vi "CommunicationTool - 副本.vi"(0 "VISA资源名称":refnum<visa-resource-name>="COM1", 1 "SN":string, 5 "通信协议名称":string, 7 "Slot":T1, 9 "DelayTime":u32=1000, 11 "error in":errorcluster, 12 "Debug":bool) -> (3 "字符串数值":bool=TRUE, 4 "响应":string="ÿÿÿÿÿÿÿÿÿÿÿÿÿÿÿÿÿÿÿÿÿÿÿÿÿÿÿ", 6 "反馈结果":bool, 10 "CMD":string, 14 "data":string, 15 "error out":errorcluster)   [LabVIEW 2013]
doc: "本范例根据用户指示，对串口执行读写操作。范例运行时可按下“写入”或“读取”按钮，以及修改“读数”。\n\n设置的串口参数必须匹配连接仪器或设备的参数。本范例中，“读数”参数可指定串口读取的字节数。如端口字节超过指定的字节数，超出部分将不会被读取。如端口字节数少于指定的字节数，将返回超时错误。\n\n本范例可扩展流控制选项以包括XON和XOFF，从而允许用户选择控制字符。同时，用户可启用或禁用中止符。部分设备需要通过终止符确定命令字符串的结束位置。部分设备将发送终止符以说明待读取数据的末端。本范例演示了缓冲区中检测到终止符时，结束“读取”操作或添加终止符至“写入”数据末端的方法。"
uses:
  SystemCode/SysControl/Slot.ctl
  <vilib>/Utility/NIReport.llb/NI_report.lvclass
  C:/Program Files/National Instruments/LabVIEW 2013/examples/Instrument IO/Serial/support/Serial - Settings.ctl
  SourceCode/GlobalValue.vi
  <vilib>/Utility/error.llb/Error Cluster From Error Code.vi
  <vilib>/addons/_office/excel.llb/Excel Get Data ([str]).vi
  <vilib>/Instr/_visa.llb/VISA Configure Serial Port (Instr).vi
  <vilib>/ErrorRing/Error Ring.xnode
  <vilib>/addons/_office/NI_ReportGenerationToolkit.lvlib
  <vilib>/Utility/NIReport.llb/Excel/NI_Excel.lvclass
panel:
  out "SerNO":string
  out "硬件版本":string
  out "终端ID":string
  out "CCID":string="PASS"
  out "生产日期":string
  out "字符串":string
  out "x-y":u32
  out "已删除的部分":u8[](array[numeric]) format="%x"
  out "读取缓冲区":string
  out "数据Hex":string[](array[string])
  out "数据ASCII":string[](array[string])
  out "数据类型":string[](array[string])
  in  "命令列表":u16(ring)=17 items=["启动自动化测试", "查询版本", "退出自动化测试", "进入待机模式", "进入工作模式", "查询ACC状态", "GPS定位查询", "GPS定位时间", "GPS可见星数", "3G通信自检", "3G信号强度", "查询网络状态", "拨号", "查询通话状态", "挂断", "外部Flash测试", "查询BAT7.2V_DET电压", "查询BAT_DET状态", "查询ANT1_0状态", "BATVCC_CTL输出低电平", "BATVCC_CTL输出高电平", "CHARGE_CTL输出低电平", "CHARGE_CTL输出高电平", "查询CHARGE_WAKE状态", "3G_PWR_CTL输出低电平", "3G_PWR_CTL输出高电平", "3G_RST输出低电平", "3G_RST输出高电平", "查询ANT1_S状态", "GPS_PWREN输出低电平", "GPS_PWREN输出高电平", "CAN通信接收", "CAN通信发送", "重启", "U_CTL输出低电平", "U_CTL输出高电平", "OBD_CTL输出低电平", "OBD_CTL输出高电平", "OBD_STB输出低电平", "OBD_STB输出高电平", "3G_EN输出低电平", "3G_EN输出高电平", "写入五菱主机条码", "写入主机条码", "读出五菱主机条码", "读出主机条码", "写入生产日期", "读出生产日期", "读出CCID", "写入终端ID", "读出终端ID", "写入硬件版本", "读出硬件版本", "查看TBC文件"]
  out "Write":bool
  out "Read":bool
  out "ConfigPath":string="C:\\Users\\dell\\Desktop\\ExcelReport.vi"
  out "Data":string
  out "DataType":string
  out "命令":string
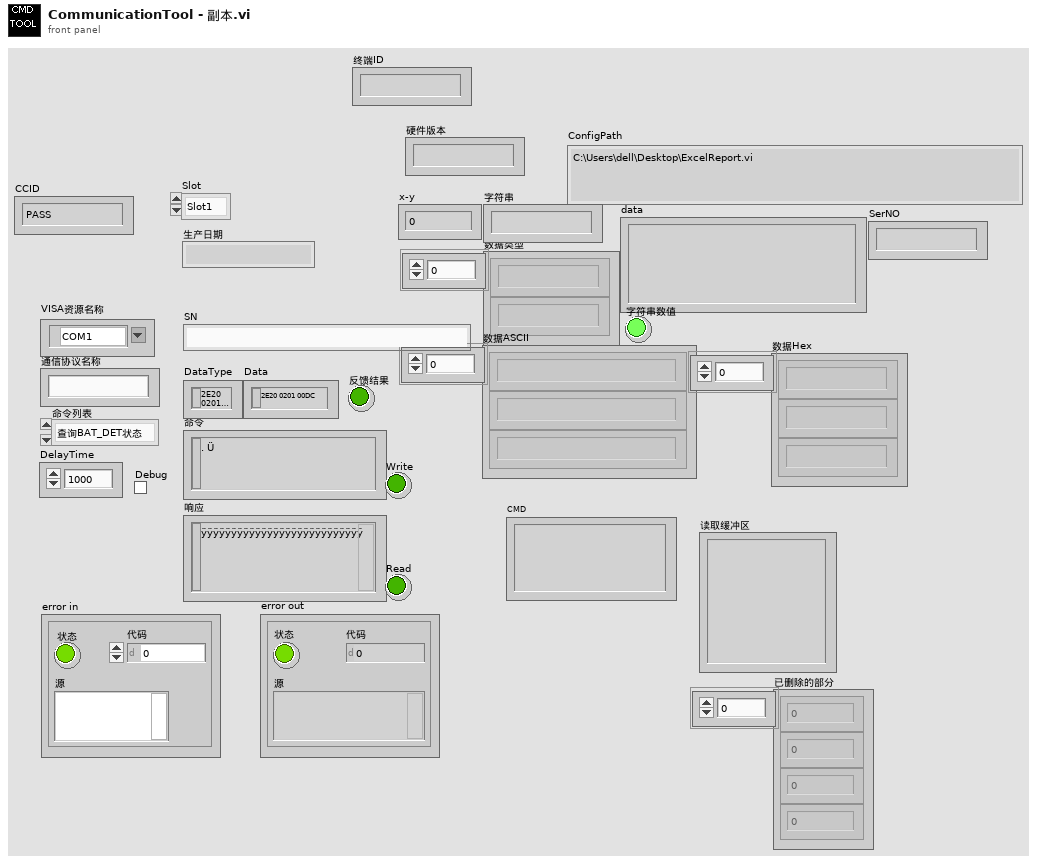
[diagram p1: front panel]
types:
  T1 = typedef "Slot.ctl" = enum16{"Slot1", "Slot2", "Slot3", "Slot4"}
  T2 = enum32{"invalid app kind", "Development System", "Run Time System", "Student Edition", "Embedded LabVIEW", "Evaluation", "Custom"}
  T3 = enum16{"maximized", "minimized", "normal", "no change"}
  T4 = enum16{"Standard Report", "HTML", "Word", "Excel"}
  T5 = typedef "Serial - Settings.ctl" = cluster{"波特率":u32, "数据比特":u16, "奇偶":enum16{"None", "Odd", "Even", "Mark", "Space"}, "停止位":u16, "流控制":u16}
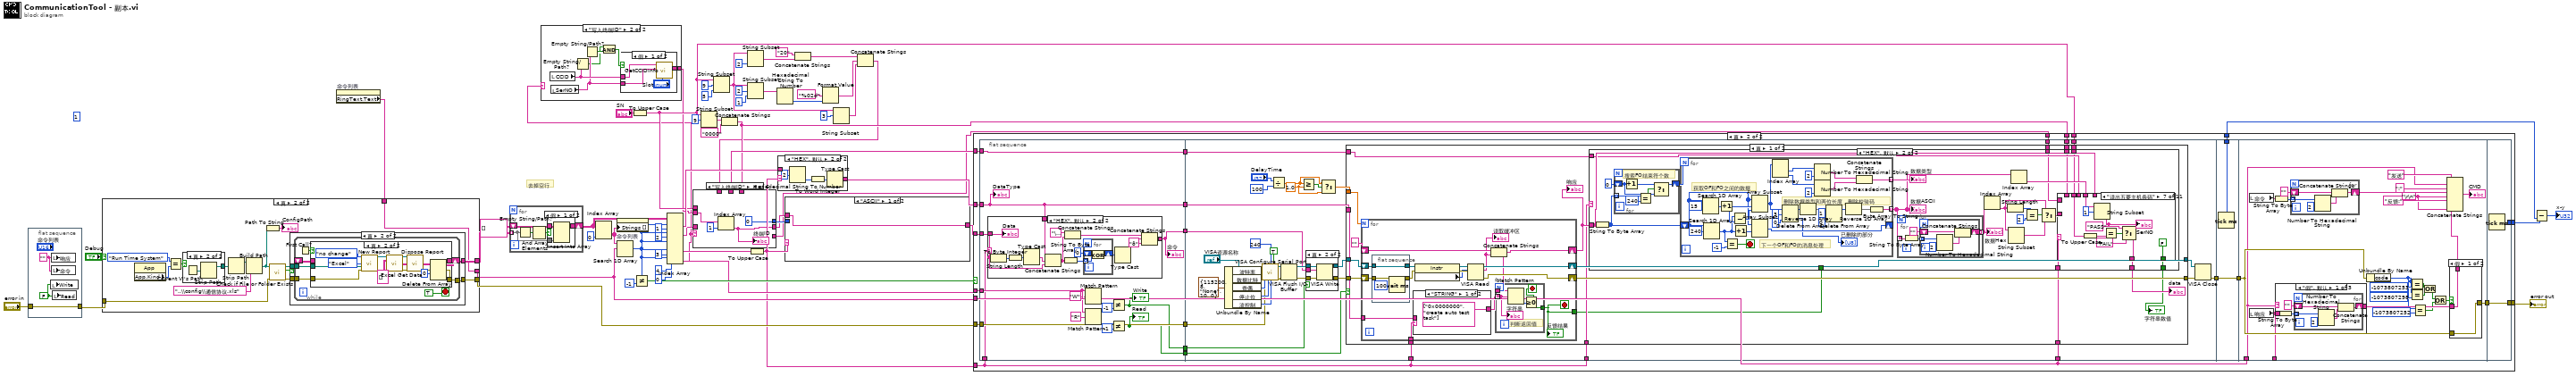
[diagram p0: block diagram]
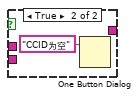
[diagram p3: hidden frame]
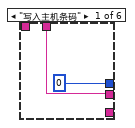
[diagram p4: hidden frame]
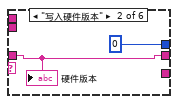
[diagram p5: hidden frame]
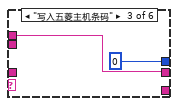
[diagram p6: hidden frame]
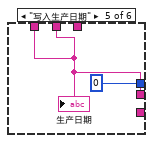
[diagram p7: hidden frame]
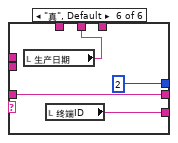
[diagram p8: hidden frame]
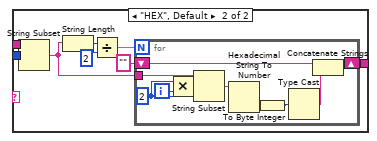
[diagram p11: hidden frame]
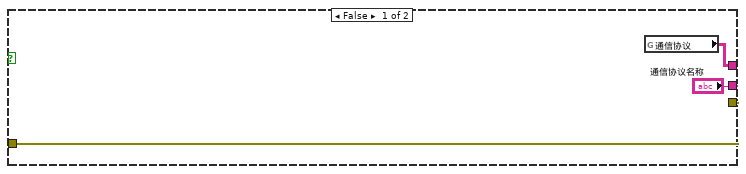
[diagram p12: hidden frame]
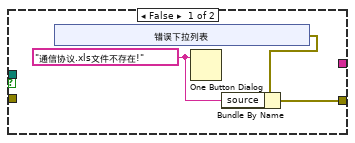
[diagram p13: hidden frame]
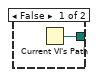
[diagram p15: hidden frame]
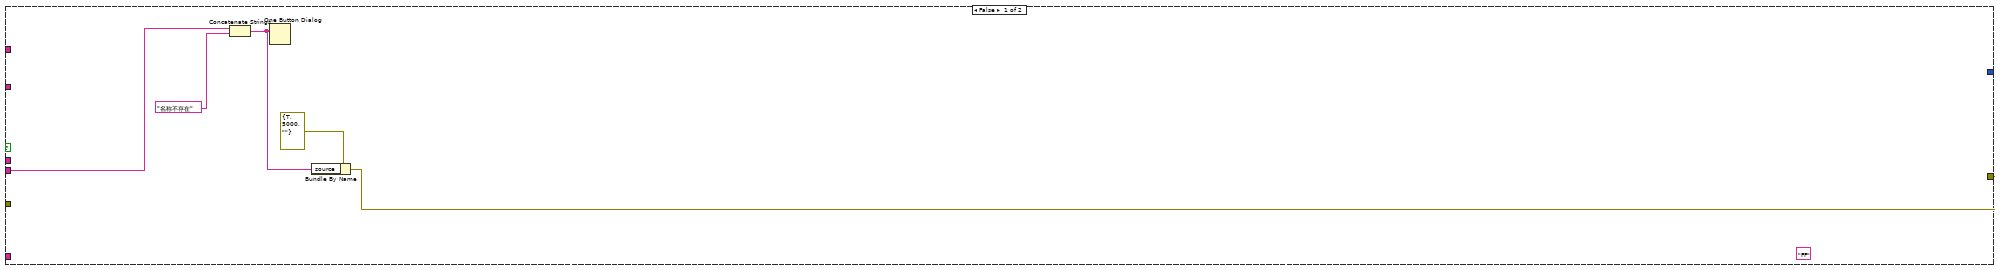
[diagram p16: hidden frame]
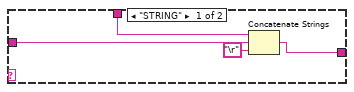
[diagram p17: hidden frame]
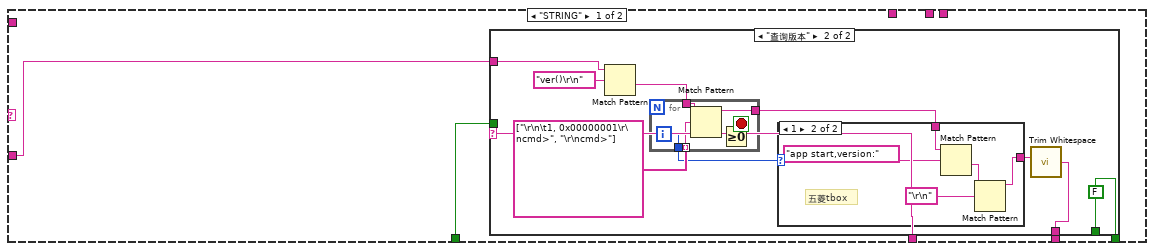
[diagram p19: hidden frame]
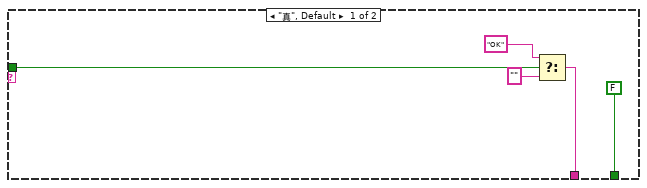
[diagram p20: hidden frame]
diagram:
  (unwired) 1
  # "去掉空行"
  n1 = flat-sequence {
    tunnel: "error in" -> [w59]
    tunnel: [w59] -> w56
    frame #0 {
      w61 = FALSE ("Read")
      w60 = "" ("响应")
      n2 = local write "Write"(w61) -> ()
      n3 = local write "响应"(w60) -> ()
      n4 = local write "命令"(w60) -> ()
      n5 = local write "Read"(w61) -> ()
    }
  }
  n6 = property on="命令列表" class="Ring (严格)"() -> ("RingText.Text"=w55:string)  [unwired: 2 in, 2 out]
  n7 = case shown="真" "Debug" {
    tunnel: [w63 w68] -> w53
    tunnel: w56 -> [w63 w67]
    tunnel: ["通信协议名称" w65] -> w44
    tunnel: [w62 w66] -> w36
    tunnel: w55 -> [_ w65]
    frame False {
      n8 = global read "GlobalValue.vi" "通信协议"() -> (w62:string[][])
    }
    frame True {
      n9 = property class="App"() -> ("App.Kind"=w77:T2)  [unwired: 2 in, 2 out]
      n10 = Equal?(x=T2."Run Time System" ("y"), y=w77) -> (x = y?=w79:bool)
      n11 = case shown="真" w79 {
        tunnel: [w113 w115] -> w78
        frame False {
          n12 = Current VI's Path() -> (path=w113:path)
        }
        frame True {
          n13 = Current VI's Path() -> (path=w114:path)
          n14 = Strip Path(path=w114) -> (stripped path=w115:path)  [unwired: 1 out]
        }
      }
      n15 = Strip Path(path=w78) -> (stripped path=w72:path)  [unwired: 1 out]
      n16 = Build Path(base path=w72, name or relative path="..\\config\\通信协议.xls" ("连接的字符串")) -> (appended path=w74:path)
      n17 = Path To String(path=w74) -> (string=→"ConfigPath":string)
      n18 = call <vilib>:"Check if File or Folder Exists.vi"("error in (no error)"=w67, "path"=w74) -> ("error out"=w69:errorcluster, "file or folder exists?"=w71:bool, "dup path"=w70:path)  [unwired: 7 out]
      n19 = case shown="真" w71 {
        tunnel: w70 -> [_ w90]
        tunnel: w69 -> [_ w89]
        tunnel: [w81 w88] -> w68
        tunnel: [_ w87] -> w66
        frame False {
          w82 = "通信协议.xls文件不存在!" ("消息")
          n20 = xnode "错误下拉列表"() -> ("错误输出"=w80:errorcluster)
          n21 = One Button Dialog(message=w82) -> ()  [unwired: 1 in, 1 out]
          n22 = Bundle By Name(cluster=w80, "source"=w82) -> (w81:errorcluster)
        }
        frame True {
          n23 = while {
            tunnel: w90 -> [w96]
            tunnel: [w95] -> w88
            tunnel: w89 -> [w94]
            shift-right: [w97] -> w87
            shift-left: _ -> [w92]
            stop <- TRUE stop-if-true
            n24 = First Call?() -> (First Call?: T/F=w91:bool)
            n25 = case shown="真" w91 {
              tunnel: [w99 w103] -> w97
              tunnel: w96 -> [_ w102]
              tunnel: [w98 w101] -> w95
              tunnel: w94 -> [w98 w100]
              tunnel: w92 -> [w99 _]
              frame False {
              }
              frame True {
                n26 = call <vilib>:"New Report.vi"("window state (normal)"=T3."no change", "report type"=T4."Excel", "template (empty)"=w102, "error in (no error)"=w100) -> ("report out"=w108:refnum<class "NI_report.lvclass">, "error out"=w109:errorcluster)  [unwired: 2 in, 8 out]
                n27 = call-poly <vilib>:"Excel Get Data.vi"("report in"=w108, "data type"=string[][] [], "error in (no error)"=w109) -> ("report out"=w105:refnum<class "NI_report.lvclass">, "data"=w110:string[][], "error out"=w104:errorcluster)  [unwired: 10 in]
                n28 = call-dynamic "Dispose Report.vi"("report in"=w105, "error in (no error)"=w104) -> ("error out"=w101:errorcluster)  [unwired: 3 in, 10 out]
                n29 = Delete From Array(array=w110, index (row)=0 ("索引 (行)")) -> (array with subset deleted=w103:string[][])  [unwired: 2 in, 1 out]
              }
            }
          }
        }
      }
    }
  }
  n30 = for {
    tunnel: w36 -> [w116] mode=indexing
    shift-right: [w119] -> w35
    shift-left: string[][] [] -> [w120]
    n31 = Empty String/Path?(string/path=w116) -> (empty?=w118:bool[])
    n32 = And Array Elements(Boolean array=w118) -> (logical AND=w117:bool)
    n33 = case shown="假" w117 {
      tunnel: w120 -> [w123 w124]
      tunnel: [w122 w124] -> w119
      tunnel: w116 -> [w121 _]
      frame False {
        n34 = Insert Into Array(array=w123, new element=w121) -> (w122:string[][])  [unwired: 2 in]
      }
      frame True {
      }
    }
  }
  n35 = Index Array(array=w35, index (col)=0 ("禁用的索引 (列)")) -> (element=w42:string[])  [unwired: 1 in]
  n36 = property on="命令列表" class="Ring (严格)"("Strings []"=w42) -> ()  [unwired: 2 in, 2 out]
  n37 = Search 1D Array(1D array=w42, element=w44) -> (index of element=w31:i32)  [unwired: 1 in]
  n38 = To Upper Case(1:"SN") -> (0:w5:string)
  n39 = Not Equal?(x=w31, y=-1) -> (x != y?=w48:bool)
  n40 = Index Array(array=w35, index (row) #1=w31, index (col) #1=1 ("索引 (列)"), index (row) #2=w31, index (col) #2=2 ("索引 (列)"), index (row) #3=w31, index (col) #3=3 ("索引 (列)"), index (row) #4=w31, index (col) #4=4 ("禁用的索引 (列)"), index (row) #5=w31, index (col) #5=0 ("禁用的索引 (列)")) -> (element #1=w47:string, element #2=w29:string, element #3=w38:string, element #4=w40:string, element #5=w1:string)
  n41 = case shown="\"写入终端ID\"" w1 {
    tunnel: [_ w130] -> w4
    frame "假", Default {
    }
    frame "写入终端ID" {
      n42 = local read "CCID"() -> (w129:string)
      n43 = local read "SerNO"() -> (w128:string)
      n44 = Empty String/Path?(string/path=w129) -> (empty?=w126:bool)
      n45 = Empty String/Path?(string/path=w128) -> (empty?=w127:bool)
      n46 = And(x=w126, y=w127) -> (x .and. y?=w125:bool)
      n47 = case shown="假" w125 {
        tunnel: [w134 _] -> w130
        tunnel: w129 -> [w132 _]
        tunnel: w128 -> [w131 _]
        frame False {
          n48 = call "GetCCIDInfo.vi"("Slot"="Slot", "SerNO"=w131, "CCID"=w132) -> ("CCID信息"=w134:string[])  [unwired: 8 in]
        }
        frame True {
          n49 = One Button Dialog(message="CCID为空" ("消息")) -> ()  [unwired: 1 in, 1 out]
        }
      }
    }
  }
  n50 = String Subset(string=w5, offset (0)=9 ("偏移量(0)")) -> (substring=w24:string)  [unwired: 1 in]
  n51 = String Subset(string=w5, offset (0)=9 ("偏移量(0)"), length (rest)=5 ("长度（剩余）")) -> (substring=w12:string)
  n52 = Concatenate Strings(w24, "0000" ("字符串")) -> (w22:string)
  n53 = String Subset(string=w12, length (rest)=2 ("长度（剩余）")) -> (substring=w19:string)  [unwired: 1 in]
  n54 = String Subset(string=w12, offset (0)=2 ("偏移量(0)"), length (rest)=1 ("长度（剩余）")) -> (substring=w14:string)
  n55 = To Upper Case(1:w38) -> (0:w34:string)
  n56 = Hexadecimal String To Number(string=w14) -> (number=w9:u32)  [unwired: 2 in, 1 out]
  n57 = case shown="\"HEX\", 默认" w34 {
    tunnel: w47 -> [w136 w139]
    tunnel: [w136 w137] -> w46
    frame "STRING" {
    }
    frame "HEX", Default {
      n58 = Hexadecimal String To Number(string=w139, offset=2 ("偏移量")) -> (number=w141:u32)  [unwired: 1 in, 1 out]
      n59 = To Word Integer(number=w141) -> (16bit integer=w138:i16)
      n60 = Type Cast(x=w138) -> (*(type *) &x=w137:string)  [unwired: 1 in]
    }
  }
  n61 = Concatenate Strings("20" ("字符串"), w19) -> (w11:string)
  n62 = Format Value(format string="%02d" ("格式字符串"), value (0)=w9) -> (output string=w7:string)  [unwired: 1 in]
  n63 = String Subset(string=w12, offset (0)=3 ("偏移量(0)")) -> (substring=w10:string)  [unwired: 1 in]
  n64 = Concatenate Strings(w11, w7, w10) -> (w6:string)
  n65 = case shown="\"写入终端ID\"" w1 {
    tunnel: w29 -> [_ w144 _ _ _ w157]
    tunnel: [w142 w144 w146 w148 w152 w157] -> w3
    tunnel: [0 ("偏移量(0)") 0 ("偏移量(0)") 0 ("偏移量(0)") 0 ("偏移量(0)") 0 ("偏移量(0)") 2 ("偏移量(0)")] -> w28
    tunnel: [_ _ _ _ w152 w155] -> w26
    tunnel: w22 -> [w142 _ _ _ _ _]
    tunnel: w6 -> [_ _ _ _ w152 _]
    tunnel: w5 -> [_ _ w146 _ _ _]
    tunnel: w4 -> [_ _ _ w150 _ _]
    tunnel: [_ _ _ _ _ w154] -> w2
    frame "写入主机条码" {
    }
    frame "写入硬件版本" {
      "硬件版本" <- w144
    }
    frame "写入五菱主机条码" {
    }
    frame "写入终端ID" {
      n66 = Index Array(array=w150, index=1 ("索引")) -> (element=w148:string)
      "终端ID" <- w148
    }
    frame "写入生产日期" {
      "生产日期" <- w152
    }
    frame "真", Default {
      n67 = local read "生产日期"() -> (w155:string)
      n68 = local read "终端ID"() -> (w154:string)
    }
  }
  n69 = case shown="\"ASCII\"" w34 {
    tunnel: [w158 w163] -> w45
    tunnel: w3 -> [w158 w162]
    tunnel: w28 -> [_ w159]
    frame "ASCII" {
    }
    frame "HEX", Default {
      n70 = String Subset(string=w162, offset (0)=w159) -> (substring=w161:string)  [unwired: 1 in]
      n71 = String Length(string=w161) -> (length=w165:i32)
      n72 = Divide(x=w165, y=2) -> (x/y=w160:dbl)
      n73 = for {
        N: w160 -> [_]
        tunnel: w161 -> [w171]
        shift-right: [w173] -> w163
        shift-left: "" -> [w172]
        i -> [w169]
        w167 = 2 ("x")
        n74 = Multiply(x=w167, y=w169) -> (x*y=w168:i32)
        n75 = String Subset(string=w171, offset (0)=w168, length (rest)=w167) -> (substring=w170:string)
        n76 = Hexadecimal String To Number(string=w170) -> (number=w176:u32)  [unwired: 2 in, 1 out]
        n77 = To Byte Integer(number=w176) -> (8bit integer=w175:i8)
        n78 = Type Cast(x=w175) -> (*(type *) &x=w174:string)  [unwired: 1 in]
        n79 = Concatenate Strings(w172, w174) -> (w173:string)
      }
    }
  }
  n80 = case shown="真" w48 {
    tunnel: w44 -> [w181 w192]
    tunnel: w46 -> [_ w203]
    tunnel: w45 -> [_ w202]
    tunnel: w53 -> [_ w201]
    tunnel: [w177 w199] -> w58
    tunnel: w40 -> [_ w198]
    tunnel: w34 -> [_ w193]
    tunnel: [_ w188] -> w54
    tunnel: [_ w187] -> w33
    tunnel: w26 -> [_ w186]
    tunnel: w22 -> [_ w184]
    tunnel: w5 -> [_ w183]
    tunnel: w2 -> [_ w182]
    frame False {
      (unwired) "FF" ("响应")
      n81 = Concatenate Strings(w181, "名称不存在" ("消息")) -> (w178:string)
      n82 = One Button Dialog(message=w178) -> ()  [unwired: 1 in, 1 out]
      n83 = Bundle By Name(cluster=errorcluster {"status"=TRUE, "code"=5000, "source"=""} ("error in 1 (no error)"), "source"=w178) -> (w177:errorcluster)
    }
    frame True {
      n84 = flat-sequence {
        tunnel: w203 -> [w206]
        tunnel: w202 -> [w208]
        tunnel: w201 -> [w218]
        tunnel: [w218] -> w200
        tunnel: w198 -> [w217]
        tunnel: [w210] -> w197
        tunnel: [w209] -> w196
        tunnel: [w207] -> w195
        tunnel: [w206] -> w194
        tunnel: w193 -> [w205]
        tunnel: w186 -> [w204]
        tunnel: [w204] -> w185
        tunnel: w200 -> [w266]
        tunnel: w197 -> [w256]
        tunnel: w196 -> [w264]
        tunnel: [w265] -> w191
        tunnel: w195 -> [w257]
        tunnel: w194 -> [w255]
        tunnel: w193 -> [w246]
        tunnel: w193 -> [w245]
        tunnel: w192 -> [w244]
        tunnel: w185 -> [w243]
        tunnel: w184 -> [w242]
        tunnel: w183 -> [w241]
        tunnel: w182 -> [w240]
        tunnel: w191 -> [w519]
        tunnel: [w519] -> w190
        tunnel: [w518] -> w187
        tunnel: w190 -> [w532]
        tunnel: w192 -> [w520]
        tunnel: [w521] -> _
        tunnel: [w533] -> w189
        tunnel: [w565] -> w199
        tunnel: w189 -> [w565]
        tunnel: [w564] -> w188
        frame #0 {
          n85 = case shown="\"HEX\", 默认" w205 {
            tunnel: w208 -> [w221 w233]
            tunnel: [w220 w227] -> w207
            tunnel: w206 -> [w222 w226]
            frame "STRING" {
              n86 = Concatenate Strings(w222, w221, "\r") -> (w220:string)
            }
            frame "HEX", Default {
              n87 = String Length(string=w233) -> (length=w224:i32)
              n88 = To Byte Integer(number=w224) -> (8bit integer=w225:i8)
              n89 = Type Cast(x=w225) -> (*(type *) &x=w223:string)  [unwired: 1 in]
              n90 = Concatenate Strings(w226, w223, w233) -> (w236:string)
              n91 = String To Byte Array(string=w236) -> (unsigned byte array=w232:u8[])
              n92 = Concatenate Strings("\u000f" ("HeadCode"), w236) -> (w229:string)
              n93 = for {
                tunnel: w232 -> [w239] mode=indexing
                shift-right: [w237] -> w230
                shift-left: u8 0 ("y") -> [w238]
                n94 = Exclusive Or(1:w239, 2:w238) -> (0:w237:u8)
              }
              n95 = Type Cast(x=w230) -> (*(type *) &x=w234:string)  [unwired: 1 in]
              n96 = Concatenate Strings(w229, w234, "ð" ("字符串")) -> (w227:string)
              "Data" <- w233
            }
          }
          "命令" <- w207
          n97 = Match Pattern(string=w217, regular expression="W" ("正则表达式")) -> (offset past match=w211:i32)  [unwired: 1 in, 3 out]
          n98 = Match Pattern(string=w217, regular expression="R" ("正则表达式")) -> (offset past match=w212:i32)  [unwired: 1 in, 3 out]
          n99 = Not Equal?(x=w211, y=-1) -> (x != y?=w210:bool)
          "Write" <- w210
          n100 = Not Equal?(x=w212, y=-1) -> (x != y?=w209:bool)
          "Read" <- w209
          "DataType" <- w206
        }
        frame #1 {
          w252 = 1.0 ("y")
          n101 = Unbundle By Name(T5 {"波特率"=115200, "数据比特"=8, "奇偶"=enum."None", "停止位"=10, "流控制"=0} ("串口设置")) -> ("波特率"=w271:u32, "数据比特"=w272:u16, "奇偶"=w273:enum16{"None", "Odd", "Even", "Mark", "Space"}, "停止位"=w274:u16, "流控制"=w267:u16)
          n102 = call-poly "VISA Configure Serial Port"("VISA resource name"="VISA资源名称", "termination char\n(0xA = '\\n' = LF)"=u8 240 ("termination char\n(0xA = '\\n' = LF)"), "Enable Termination\nChar (T)"=TRUE ("Enable Termination\nChar (T)"), "baud rate (9600)"=w271, "data bits (8)"=w272, "parity (0:none)"=w273, "error in (no error)"=w266, "stop bits (10: 1 bit)"=w274, "flow control (0:none)"=w267) -> ("VISA resource name out"=w261:refnum<visa-resource-name>, "error out"=w262:errorcluster)  [unwired: 1 in, 4 out]
          n103 = Divide(x="DelayTime", y=u32 100) -> (x/y=w251:dbl)
          n104 = VISA Flush I/O Buffer(VISA resource name=w261, error in (no error)=w262) -> (VISA resource name out=w260:refnum<visa-resource-name>, error out=w259:errorcluster)  [unwired: 1 in]
          n105 = Greater Or Equal?(x=w251, y=w252) -> (x >= y?=w250:bool)
          n106 = case shown="真" w256 {
            tunnel: w260 -> [w277 w282]
            tunnel: [w277 w281] -> w254
            tunnel: [w276 w280] -> w253
            tunnel: w259 -> [w276 w279]
            tunnel: w257 -> [_ w278]
            frame False {
            }
            frame True {
              n107 = VISA Write(VISA resource name=w282, write buffer=w278, error in (no error)=w279) -> (VISA resource name out=w281:refnum<visa-resource-name>, error out=w280:errorcluster)  [unwired: 1 out]
            }
          }
          n108 = Select(t=w251, s=w250, f=w252) -> (s? t:f=w247:dbl)
          n109 = case shown="真" w264 {
            tunnel: [w299 w517] -> w268
            tunnel: w254 -> [w298 w517]
            tunnel: [w300 w516] -> w269
            tunnel: w253 -> [w297 w516]
            tunnel: w255 -> [w294 _]
            tunnel: w247 -> [w293 _]
            tunnel: w246 -> [w292 _]
            tunnel: w245 -> [w291 _]
            tunnel: w244 -> [w289 _]
            tunnel: w243 -> [w286 _]
            tunnel: w242 -> [w285 _]
            tunnel: w241 -> [w284 _]
            tunnel: w240 -> [w283 _]
            frame True {
              n110 = for {
                N: w293 -> [_]
                shift-right: [w500] -> w300
                shift-left: w297 -> [w489]
                shift-right: [w487] -> w295
                shift-left: "" ("read buffer") -> [w495]
                shift-right: [w499] -> w299
                shift-left: w298 -> [w488]
                tunnel: w294 -> [w492]
                tunnel: w292 -> [w486]
                tunnel: [w485] -> w290
                stop <- w485 stop-if-true
                n111 = flat-sequence {
                  tunnel: w489 -> [w515]
                  tunnel: [w515] -> w490
                  tunnel: [w514] -> w491
                  tunnel: w488 -> [w514]
                  frame #0 {
                    n112 = Wait (ms)(milliseconds to wait=u32 100 ("等待时间（毫秒）")) -> ()  [unwired: 1 out]
                  }
                }
                n113 = case shown="\"STRING\"" w486 {
                  tunnel: [string[] ["0x0000000", "create auto test task"] w506] -> w494
                  tunnel: w492 -> [_ w512]
                  frame "STRING" {
                  }
                  frame "HEX", Default {
                    n114 = String Subset(string=w512, offset (0)=1 ("偏移量(0)")) -> (substring=w509:string)  [unwired: 1 in]
                    n115 = Concatenate Strings("\u000f€" ("正则表达式"), w509) -> (w508:string)
                    n116 = call "SearchSpecialChar.vi"("正则表达式"=w508) -> ("字符串"=w507:string)
                    n117 = Build Array(w507) -> (w506:string[])
                  }
                }
                n118 = property class="Instr"(reference=w491, error in=w490) -> (reference out=w498:refnum<visa-resource-name>, error out=w497:errorcluster, "Serial Settings:Number of Bytes at Serial Port"=w496:u32)
                n119 = VISA Read(VISA resource name=w498, byte count=w496, error in (no error)=w497) -> (VISA resource name out=w499:refnum<visa-resource-name>, read buffer=w493:string, error out=w500:errorcluster)  [unwired: 1 out]
                "读取缓冲区" <- w493
                n120 = Concatenate Strings(w495, w493) -> (w487:string)
                n121 = for {
                  tunnel: w494 -> [w501] mode=indexing
                  tunnel: w487 -> [w503]
                  tunnel: [w502] -> w485
                  stop <- w502 stop-if-true
                  # "判断返回值"
                  n122 = Match Pattern(string=w503, regular expression=w501) -> (offset past match=w504:i32)  [unwired: 1 in, 3 out]
                  n123 = Greater Or Equal To 0?(x=w504) -> (x >= 0?=w502:bool)
                  "字符串" <- w501
                }
                "反馈结果" <- w485
              }
              "响应" <- w295
              n124 = case shown="\"HEX\", 默认" w291 {
                tunnel: w295 -> [w304 w338]
                tunnel: w290 -> [w301 _]
                tunnel: w289 -> [w305 w346]
                tunnel: [w303 w345] -> w288
                tunnel: [w302 w344] -> w287
                tunnel: w286 -> [_ w335]
                tunnel: w285 -> [_ w334]
                tunnel: w284 -> [_ w333]
                tunnel: w283 -> [_ w332]
                frame "STRING" {
                  n125 = case shown="\"查询版本\"" w305 {
                    tunnel: [w306 w311] -> w303
                    tunnel: [FALSE FALSE] -> w302
                    tunnel: w304 -> [_ w318]
                    tunnel: w301 -> [w307 _]
                    frame "真", Default {
                      n126 = Select(t="OK", s=w307, f="") -> (s? t:f=w306:string)
                    }
                    frame "查询版本" {
                      n127 = Match Pattern(string=w318, regular expression="ver()\r\n" ("正则表达式")) -> (after substring=w316:string)  [unwired: 1 in, 3 out]
                      n128 = for {
                        tunnel: w316 -> [w331]
                        tunnel: [w330] -> w313
                        tunnel: string[] ["\r\n\t1, 0x00000001\r\ncmd>", "\r\ncmd>"] -> [w327] mode=indexing
                        tunnel: [w326] -> w314
                        i -> [w326]
                        stop <- w328 stop-if-true
                        n129 = Match Pattern(string=w331, regular expression=w327) -> (before substring=w330:string, offset past match=w329:i32)  [unwired: 1 in, 2 out]
                        n130 = Greater Or Equal To 0?(x=w329) -> (x >= 0?=w328:bool)
                      }
                      n131 = case shown="1" w314 {
                        tunnel: [w320 w321] -> w312
                        tunnel: w313 -> [w320 w325]
                        frame 0, Default {
                          # "海马tbox"
                        }
                        frame 1 {
                          # "五菱tbox"
                          n132 = Match Pattern(string=w325, regular expression="app start,version:" ("正则表达式")) -> (after substring=w323:string)  [unwired: 1 in, 3 out]
                          n133 = Match Pattern(string=w323, regular expression="\r\n" ("正则表达式")) -> (before substring=w321:string)  [unwired: 1 in, 3 out]
                        }
                      }
                      n134 = call <vilib>:"Trim Whitespace.vi"("string"=w312) -> ("trimmed string"=w311:string)  [unwired: 1 in]
                    }
                  }
                }
                frame "HEX", Default {
                  n135 = String To Byte Array(string=w338) -> (unsigned byte array=w343:u8[])
                  n136 = for {
                    tunnel: w343 -> [w367] mode=indexing
                    shift-right: [w363] -> w341
                    shift-left: 0 ("y") -> [w362]
                    # "搜索FO结束符个数"
                    n137 = Increment(x=w362) -> (x+1=w364:i32)
                    n138 = Equal?(x=w367, y=u8 240) -> (x = y?=w365:bool)
                    n139 = Select(t=w364, s=w365, f=w362) -> (s? t:f=w363:i32)
                  }
                  n140 = for {
                    N: w341 -> [_]
                    shift-right: [w390] -> _
                    shift-left: w343 -> [w391]
                    tunnel: [w374] -> w337 mode=indexing
                    tunnel: [w370] -> w340 mode=indexing
                    stop <- w388 stop-if-true
                    # "删除数据类型和两位长度，删除校验码"
                    # "下一个OF和FO的消息处理"
                    # "获取OF和FO之间的数据"
                    n141 = Search 1D Array(1D array=w391, element=u8 15 ("元素")) -> (index of element=w393:i32)  [unwired: 1 in]
                    n142 = Search 1D Array(1D array=w391, element=u8 240 ("元素")) -> (index of element=w386:i32)  [unwired: 1 in]
                    n143 = Increment(x=w393) -> (x+1=w392:i32)
                    n144 = Equal?(x=w386, y=-1) -> (x = y?=w388:bool)
                    n145 = Subtract(x=w386, y=w392) -> (x-y=w394:i32)
                    n146 = Increment(x=w386) -> (x+1=w387:i32)
                    n147 = Array Subset(array=w391, index=w392, length=w394) -> (w383:u8[])
                    n148 = Array Subset(array=w391, index=w387) -> (w390:u8[])  [unwired: 1 in]
                    n149 = Index Array(array=w383) -> (element #1=w384:u8, element #2=w373:u8)  [unwired: 2 in]
                    n150 = Delete From Array(array=w383, length=3 ("长度"), index=0 ("索引")) -> (deleted portion=→"已删除的部分":u8[], array with subset deleted=w380:u8[])
                    n151 = Reverse 1D Array(array=w380) -> (reversed array=w379:u8[])
                    n152 = Number To Hexadecimal String(1:i16 2 ("宽度(-)"), 2:w384) -> (0:w371:string)
                    n153 = Number To Hexadecimal String(1:i16 2 ("宽度(-)"), 2:w373) -> (0:w372:string)
                    n154 = Delete From Array(array=w379, length=1 ("长度"), index=0 ("索引")) -> (array with subset deleted=w376:u8[])  [unwired: 1 out]
                    n155 = Reverse 1D Array(array=w376) -> (reversed array=w375:u8[])
                    n156 = Concatenate Strings(w371, w372) -> (w370:string)
                    n157 = Byte Array To String(unsigned byte array=w375) -> (string=w374:string)
                  }
                  "数据类型" <- w340
                  "数据ASCII" <- w337
                  n158 = for {
                    tunnel: w337 -> [w356] mode=indexing
                    tunnel: [w353] -> w339 mode=indexing
                    n159 = String To Byte Array(string=w356) -> (unsigned byte array=w354:u8[])
                    n160 = for {
                      tunnel: w354 -> [w361] mode=indexing
                      shift-right: [w359] -> w353
                      shift-left: "" -> [w358]
                      n161 = Number To Hexadecimal String(1:i16 2 ("宽度(-)"), 2:w361) -> (0:w360:string)
                      n162 = Concatenate Strings(w358, w360) -> (w359:string)
                    }
                  }
                  "数据Hex" <- w339
                  n163 = Index Array(array=w339) -> (element=w349:string)  [unwired: 1 in]
                  n164 = String Length(string=w349) -> (length=w352:i32)
                  n165 = String Subset(string=w349) -> (substring=w348:string)  [unwired: 2 in]
                  n166 = Index Array(array=w337) -> (element=w336:string)  [unwired: 1 in]
                  n167 = Equal?(x=w352, y=2) -> (x = y?=w350:bool)
                  n168 = Select(t=w349, s=w350, f=w348) -> (s? t:f=w347:string)
                  n169 = case shown="\"读出五菱主机条码\"" w346 {
                    tunnel: w347 -> [w399 w412 w416 w419 _ _ _ _ _ _ _]
                    tunnel: [w398 w408 w414 w420 w425 w433 w444 w450 w461 w471 w480] -> w345
                    tunnel: [TRUE TRUE TRUE FALSE TRUE FALSE FALSE FALSE FALSE FALSE FALSE] -> w344
                    tunnel: w338 -> [_ _ _ _ w429 _ _ _ _ _ _]
                    tunnel: w336 -> [_ _ _ _ _ w437 w441 w458 w465 w468 w478]
                    tunnel: w335 -> [_ _ _ _ _ _ _ _ w460 _ _]
                    tunnel: w334 -> [_ _ _ _ _ w431 _ _ _ _ _]
                    tunnel: w333 -> [_ _ _ _ _ _ w442 _ _ _ _]
                    tunnel: w332 -> [_ _ _ _ _ _ _ _ _ w470 _]
                    frame "查询BAT7.2V_DET电压" {
                      n170 = Hexadecimal String To Number(string=w399) -> (number=w402:u32)  [unwired: 2 in, 1 out]
                      n171 = Divide(x=w402, y=u32 1000) -> (x/y=w400:dbl)
                      n172 = Number To Fractional String(number=w400) -> (F-format string=w398:string)  [unwired: 3 in]
                    }
                    frame "查询BAT_DET状态" {
                      n173 = Hexadecimal String To Number(string=w412) -> (number=w410:u32)  [unwired: 2 in, 1 out]
                      n174 = Multiply(x=w410, y=u32 11) -> (x*y=w409:u32)
                      n175 = Divide(x=w409, y=u32 1000) -> (x/y=w405:dbl)
                      n176 = Add(x=w405, y=0.3) -> (x+y=w403:dbl)
                      n177 = Number To Fractional String(number=w403) -> (F-format string=w408:string)  [unwired: 3 in]
                    }
                    frame "加速度传感器返回数据1" {
                      n178 = Hexadecimal String To Number(string=w416) -> (number=w415:u32)  [unwired: 2 in, 1 out]
                      n179 = Number To Decimal String(number=w415) -> (decimal integer string=w414:string)  [unwired: 1 in]
                    }
                    frame "真", Default {
                      n180 = Empty String/Path?(string/path=w419) -> (empty?=w418:bool)
                      n181 = case shown="假" w418 {
                        tunnel: [w422 ""] -> w420
                        tunnel: w419 -> [w421 _]
                        frame False {
                          n182 = Concatenate Strings("0x" ("字符串"), w421) -> (w422:string)
                        }
                        frame True {
                        }
                      }
                    }
                    frame "查询版本" {
                      n183 = Match Pattern(string=w429, regular expression="ver()\r\n" ("正则表达式")) -> (after substring=w427:string)  [unwired: 1 in, 3 out]
                      n184 = Match Pattern(string=w427, regular expression="\r\n\t1, 0x00000001\r\ncmd>" ("正则表达式")) -> (before substring=w425:string)  [unwired: 1 in, 3 out]
                    }
                    frame "读出主机条码" {
                      n185 = To Upper Case(1:w431) -> (0:w432:string)
                      n186 = Equal?(x=w437, y=w432) -> (x = y?=w436:bool)
                      n187 = Select(t="PASS" ("string"), s=w436, f="FAIL") -> (s? t:f=w433:string)
                    }
                    frame "读出五菱主机条码" {
                      n188 = To Upper Case(1:w442) -> (0:w443:string)
                      n189 = String Subset(string=w441, offset (0)=1 ("偏移量(0)")) -> (substring=w439:string)  [unwired: 1 in]
                      "SerNO" <- w439
                      n190 = Equal?(x=w439, y=w443) -> (x = y?=w447:bool)
                      n191 = Select(t="PASS" ("string"), s=w447, f="FAIL") -> (s? t:f=w444:string)
                    }
                    frame "读出CCID" {
                      n192 = String Subset(string=w458, offset (0)=1 ("偏移量(0)")) -> (substring=w456:string)  [unwired: 1 in]
                      n193 = To Upper Case(1:w456) -> (0:w449:string)
                      "CCID" <- w449
                      n194 = String Length(string=w449) -> (length=w453:i32)
                      n195 = Equal?(x=w453, y=20) -> (x = y?=w451:bool)
                      n196 = Select(t="PASS" ("string"), s=w451, f="FAIL") -> (s? t:f=w450:string)
                    }
                    frame "读出生产日期" {
                      n197 = Equal?(x=w465, y=w460) -> (x = y?=w464:bool)
                      n198 = Select(t="PASS" ("string"), s=w464, f="FAIL") -> (s? t:f=w461:string)
                    }
                    frame "读出终端ID" {
                      n199 = String Subset(string=w468, offset (0)=1 ("偏移量(0)")) -> (substring=w467:string)  [unwired: 1 in]
                      n200 = Equal?(x=w467, y=w470) -> (x = y?=w474:bool)
                      n201 = Select(t="PASS" ("string"), s=w474, f="FAIL") -> (s? t:f=w471:string)
                    }
                    frame "读出硬件版本" {
                      n202 = local read "硬件版本"() -> (w476:string)
                      n203 = String Subset(string=w478, offset (0)=1 ("偏移量(0)")) -> (substring=w477:string)  [unwired: 1 in]
                      n204 = Equal?(x=w477, y=w476) -> (x = y?=w483:bool)
                      n205 = Select(t="PASS" ("string"), s=w483, f="FAIL") -> (s? t:f=w480:string)
                    }
                  }
                }
              }
              "data" <- w288
              "字符串数值" <- w287
            }
            frame False {
            }
          }
          n206 = VISA Close(VISA resource name=w268, error in (no error)=w269) -> (error out=w265:errorcluster)
        }
        frame #2 {
          n207 = Tick Count (ms)() -> (millisecond timer value=w518:u32)
        }
        frame #3 {
          w540 = "\r\n"
          n208 = local read "命令"() -> (w536:string)
          n209 = local read "响应"() -> (w521:string)
          n210 = String To Byte Array(string=w536) -> (unsigned byte array=w537:u8[])
          n211 = case shown="\"假\", 默认" w520 {
            tunnel: [w545 w553 w554] -> w531
            tunnel: w521 -> [w544 w553 w554]
            frame "假", Default {
              n212 = String To Byte Array(string=w544) -> (unsigned byte array=w547:u8[])
              n213 = for {
                tunnel: w547 -> [w552] mode=indexing
                shift-right: [w550] -> w545
                shift-left: "" -> [w549]
                n214 = Number To Hexadecimal String(1:i16 2 ("宽度(-)"), 2:w552) -> (0:w551:string)
                n215 = Concatenate Strings(w549, w551) -> (w550:string)
              }
            }
            frame "启动自动化测试" {
            }
            frame "查询版本" {
            }
          }
          n216 = for {
            tunnel: w537 -> [w563] mode=indexing
            shift-right: [w561] -> w535
            shift-left: "" -> [w560]
            n217 = Number To Hexadecimal String(1:i16 2 ("宽度(-)"), 2:w563) -> (0:w562:string)
            n218 = Concatenate Strings(w560, w562) -> (w561:string)
          }
          n219 = Unbundle By Name(w532) -> ("code"=w527:i32)
          n220 = Equal?(x=w527, y=-1073807253) -> (x = y?=w528:bool)
          n221 = Equal?(x=w527, y=-1073807298) -> (x = y?=w525:bool)
          n222 = Equal?(x=w527, y=-1073807252) -> (x = y?=w522:bool)
          n223 = Or(x=w528, y=w525) -> (x .or. y?=w523:bool)
          n224 = Or(x=w523, y=w522) -> (x .or. y?=w524:bool)
          n225 = case shown="假" w524 {
            tunnel: [w556 errorcluster {"status"=FALSE, "code"=0, "source"=""} ("t")] -> w533
            tunnel: w532 -> [w556 _]
            tunnel: w531 -> [w555 _]
            tunnel: [w555 ""] -> w530
            frame False {
            }
            frame True {
            }
          }
          n226 = Concatenate Strings("发送" ("字符串"), w520, ":" ("字符串"), w535, w540, "反馈:" ("字符串"), w530, w540) -> (→"CMD":string)
        }
        frame #4 {
          n227 = Tick Count (ms)() -> (millisecond timer value=w564:u32)
        }
      }
    }
  }
  "error out" <- w58
  n228 = Subtract(x=w54, y=w33) -> (x-y=→"x-y":u32)
